vi "steady_state.vi"(1 "Beta":dbl, 2 "Alpha":dbl, 3 "C":dbl, 4 "Physical constants":T1) -> (0 "Steady state":dbl)   [LabVIEW 2015]
uses:
  physical_constants.ctl
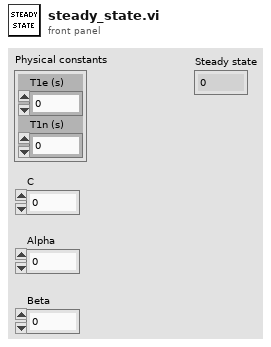
[diagram p1: front panel]
types:
  T1 = typedef "physical_constants.ctl" = cluster{"T1e (s)":dbl, "T1n (s)":dbl}
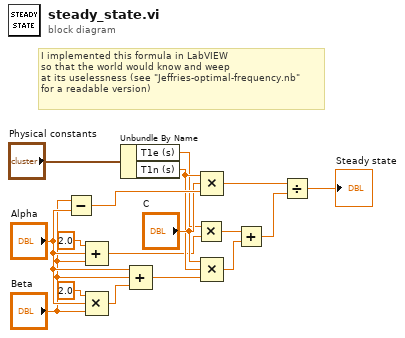
[diagram p0: block diagram]
diagram:
  # "I implemented this formula in LabVIEW\nso that the world would know and weep\nat its uselessness (see \"Jeffries-optimal-frequency.nb\"\nfor a readable version)"
  n1 = Subtract(x="Beta", y="Alpha") -> (x-y=w16:dbl)
  n2 = Compound Arithmetic op=ADD(2.0 ("value"), "Alpha", "Beta") -> (w4:dbl)
  n3 = Compound Arithmetic op=MULTIPLY(2.0 ("value"), "Alpha", "Beta") -> (w8:dbl)
  n4 = Unbundle By Name("Physical constants") -> ("T1e (s)"=w5:dbl, "T1n (s)"=w10:dbl)
  n5 = Compound Arithmetic op=ADD("Alpha", "Beta", w8) -> (w7:dbl)
  n6 = Multiply(x=w5, y=w4) -> (x*y=w6:dbl)
  n7 = Compound Arithmetic op=MULTIPLY(w10, "C", w16) -> (w15:dbl)
  n8 = Compound Arithmetic op=MULTIPLY("C", w10, w7) -> (w12:dbl)
  n9 = Add(x=w6, y=w12) -> (x+y=w14:dbl)
  n10 = Divide(x=w15, y=w14) -> (x/y=→"Steady state":dbl)
